vi "Test SWIR Camera.vi"(8 "error in (no error)":errorcluster) -> (0 "error out":errorcluster)   [LabVIEW 2018]
uses:
  <vilib>/vision/driver/IMAQdx.llb/IMAQdx Attribute Type.ctl
  <vilib>/vision/driver/IMAQdx.llb/IMAQdx Camera Control Mode.ctl
  82cda5bc-cbb3-4d55-9bbe-1a30e1cf78ab.vi
  <vilib>/Utility/file.llb/Write Delimited Spreadsheet (string).vi
  <vilib>/vision/driver/NI_Vision_Acquisition_Software.lvlib
  <resource>/objmgr/imaqdx.rc
panel:
  out "ValueU32":u32
  out "EnumStrings[]":string[](array[string])
  out "EnumValues[]":u32[](array[numeric])
  out "ValueString":string
  out "Array":string[](array[string])=["CameraAttributes::DeviceControl::DeviceInformationCommon::DeviceFirmwareRelease::DeviceFirmwareReleaseMajor", "CameraAttributes::DeviceControl::DeviceInformationCommon::DeviceFirmwareRelease::DeviceFirmwareReleaseMinor", "CameraAttributes::DeviceControl::DeviceInformationCommon::DeviceFirmwareRelease::DeviceFirmwareReleaseBuild", "CameraAttributes::DeviceControl::DeviceInformationCommon::DeviceApplicationRelease::DeviceAppReleaseMajor", "CameraAttributes::DeviceControl::DeviceInformationCommon::DeviceApplicationRelease::DeviceAppReleaseMinor", "CameraAttributes::DeviceControl::DeviceInformationCommon::DeviceApplicationRelease::DeviceAppReleaseBuild", "CameraAttributes::DeviceControl::DeviceInformationCommon::DeviceXMLRelease::DeviceXMLReleaseMajor", "CameraAttributes::DeviceControl::DeviceInformationCommon::DeviceXMLRelease::DeviceXMLReleaseMinor", "CameraAttributes::DeviceControl::DeviceInformationCommon::DeviceXMLRelease::DeviceXMLReleaseBuild", "AcquisitionAttributes::AdvancedEthernet::BandwidthControl::ActualPeakBandwidth", "AcquisitionAttributes::AdvancedEthernet::BandwidthControl::DesiredPeakBandwidth", "AcquisitionAttributes::AdvancedEthernet::Controller::DestinationMode", "AcquisitionAttributes::AdvancedEthernet::Controller::DestinationMulticastAddress", "AcquisitionAttributes::AdvancedEthernet::EventParameters::MaxOutstandingEvents", "AcquisitionAttributes::AdvancedEthernet::FirewallTraversal::Enabled", "AcquisitionAttributes::AdvancedEthernet::FirewallTraversal::KeepAliveTime", "AcquisitionAttributes::AdvancedEthernet::FirewallTraversal::Supported", "AcquisitionAttributes::AdvancedEthernet::ResendParameters::MaxResendsPerPacket", "AcquisitionAttributes::AdvancedEthernet::ResendParameters::MemoryWindowSize", "AcquisitionAttributes::AdvancedEthernet::ResendParameters::MissingPacketTimeout", "AcquisitionAttributes::AdvancedEthernet::ResendParameters::NewPacketTimeout", "AcquisitionAttributes::AdvancedEthernet::ResendParameters::ResendBatchingPercentage", "AcquisitionAttributes::AdvancedEthernet::ResendParameters::ResendResponseTimeout", "AcquisitionAttributes::AdvancedEthernet::ResendParameters::ResendThresholdPercentage", "AcquisitionAttributes::AdvancedEthernet::ResendParameters::ResendTimerResolution", "AcquisitionAttributes::AdvancedEthernet::ResendParameters::ResendsEnabled", "AcquisitionAttributes::AdvancedEthernet::TestPacketParameters::MaxTestPacketRetries", "AcquisitionAttributes::AdvancedEthernet::TestPacketParameters::TestPacketEnabled", "AcquisitionAttributes::AdvancedEthernet::TestPacketParameters::TestPacketTimeout", "CameraAttributes::DeviceControl::CoolingControl::CoolingMode", "CameraAttributes::DeviceControl::CoolingControl::CoolingTargetTemperature", "CameraAttributes::DeviceControl::CoolingControl::CoolingPower", "CameraAttributes::DeviceControl::CoolingControl::CoolingMaximalPower", "CameraAttributes::DeviceControl::CoolingControl::CoolingActualPower", "CameraAttributes::DeviceControl::CoolingControl::CoolingTargetTemperatureReached", "CameraAttributes::DeviceControl::DeviceInformationCommon::DeviceVendorName", "CameraAttributes::DeviceControl::DeviceInformationCommon::DeviceModelName", "CameraAttributes::DeviceControl::DeviceInformationCommon::DeviceManufacturerInfo", "CameraAttributes::DeviceControl::DeviceInformationCommon::DeviceVersion", "CameraAttributes::DeviceControl::DeviceInformationCommon::DeviceID", "CameraAttributes::DeviceControl::DeviceInformationCommon::DeviceUserID", "CameraAttributes::DeviceControl::DeviceInformationCommon::DeviceScanType", "CameraAttributes::AcquisitionControl::TriggerInControl::TriggerInMode", "CameraAttributes::AcquisitionControl::TriggerInControl::TriggerInEnable", "CameraAttributes::AcquisitionControl::TriggerInControl::TriggerInSensitivity", "CameraAttributes::AcquisitionControl::TriggerInControl::TriggerInPolarity", "CameraAttributes::AcquisitionControl::TriggerInControl::TriggerInDelay", "CameraAttributes::AcquisitionControl::TriggerInControl::TriggerInSkip", "CameraAttributes::AcquisitionControl::TriggerOutControl::TriggerOutEnable", "CameraAttributes::AcquisitionControl::TriggerOutControl::TriggerOutSource", "CameraAttributes::AcquisitionControl::TriggerOutControl::TriggerOutPolarity", "CameraAttributes::AcquisitionControl::TriggerOutControl::TriggerOutDelay", "CameraAttributes::AcquisitionControl::TriggerOutControl::TriggerOutWidth", "CameraAttributes::ImageProcessingControl::AutoGainControl::OffsetControl", "CameraAttributes::ImageProcessingControl::AutoGainControl::GainControl", "CameraAttributes::ImageProcessingControl::AutoGainControl::AutoModeUpdate", "CameraAttributes::ImageProcessingControl::AutoGainControl::OffsetUsed", "CameraAttributes::ImageProcessingControl::AutoGainControl::GainUsed", "CameraAttributes::ImageProcessingControl::AutoGainControl::ManualModeControl::ManualModeOffset", "CameraAttributes::ImageProcessingControl::AutoGainControl::ManualModeControl::ManualModeGain", "CameraAttributes::ImageProcessingControl::AutoGainControl::AutoModeControl::AutoModeOutputHistogramMidpoint", "CameraAttributes::ImageProcessingControl::AutoGainControl::AutoModeControl::AutoModeMaximalGain", "CameraAttributes::ImageProcessingControl::AutoGainControl::AutoModeControl::AutoModeRegulationSpeed", "CameraAttributes::ImageProcessingControl::AutoGainControl::OutliersControl::OutliersExpressedAs", "CameraAttributes::ImageProcessingControl::AutoGainControl::OutliersControl::OutliersDark", "CameraAttributes::ImageProcessingControl::AutoGainControl::OutliersControl::OutliersBright", "CameraAttributes::ImageProcessingControl::AutoGainControl::OutliersControl::OutliersBrightDisplayColor", "CameraAttributes::ImageProcessingControl::AutoGainControl::InputHistogramControl::InputHistogramBegin", "CameraAttributes::ImageProcessingControl::AutoGainControl::InputHistogramControl::InputHistogramMidpoint", "CameraAttributes::ImageProcessingControl::AutoGainControl::InputHistogramControl::InputHistogramEnd", "CameraAttributes::TransportLayer::GevVersion::GevVersionMajor", "CameraAttributes::TransportLayer::GevVersion::GevVersionMinor", "CameraAttributes::TransportLayer::GevMACAddress::GevMACAddressHigh", "CameraAttributes::TransportLayer::GevMACAddress::GevMACAddressLow", "CameraAttributes::TransportLayer::GevTimestamp::GevTimestampTickFrequency", "CameraAttributes::TransportLayer::GevTimestamp::GevTimestampControl::GevTimestampControlReset", "AcquisitionAttributes::AdvancedEthernet::GigEDriverType", "AcquisitionAttributes::AdvancedGenicam::CommandTimeout", "AcquisitionAttributes::AdvancedGenicam::EventsEnabled", "AcquisitionAttributes::AdvancedGenicam::EventsSupported", "AcquisitionAttributes::AdvancedGenicam::IgnoreCameraValidationErrors", "AcquisitionAttributes::Bayer::Algorithm", "AcquisitionAttributes::Bayer::GainB", "AcquisitionAttributes::Bayer::GainG", "AcquisitionAttributes::Bayer::GainR", "AcquisitionAttributes::Bayer::Pattern", "AcquisitionAttributes::ChunkDataDecoding::ChunkDataDecodingEnabled", "AcquisitionAttributes::ChunkDataDecoding::MaximumChunkCopySize", "CameraAttributes::DeviceControl::DeviceVTestGVoltage", "CameraAttributes::DeviceControl::DeviceDetSubVoltage", "CameraAttributes::DeviceControl::DeviceVcmVoltage", "CameraAttributes::DeviceControl::DeviceCtiaRefVoltage", "CameraAttributes::DeviceControl::DeviceROICBiasCurrent", "CameraAttributes::DeviceControl::DeviceGain", "CameraAttributes::DeviceControl::DeviceTemperature", "CameraAttributes::DeviceControl::DeviceBoardTemperature", "CameraAttributes::AcquisitionControl::AcquisitionMode", "CameraAttributes::AcquisitionControl::ExposureTimeAbs", "CameraAttributes::AcquisitionControl::IntegrationMode", "CameraAttributes::AcquisitionControl::MinimumFrameTime", "CameraAttributes::AcquisitionControl::SoftwareTrigger", "CameraAttributes::AcquisitionControl::TriggerDirection", "CameraAttributes::ImageFormatControl::WidthMax", "CameraAttributes::ImageFormatControl::HeightMax", "CameraAttributes::ImageFormatControl::Width", "CameraAttributes::ImageFormatControl::Height", "CameraAttributes::ImageFormatControl::OffsetX", "CameraAttributes::ImageFormatControl::OffsetY", "CameraAttributes::ImageFormatControl::ReverseX", "CameraAttributes::ImageFormatControl::ReverseY", "CameraAttributes::ImageFormatControl::PixelFormat", "CameraAttributes::ImageFormatControl::FooterEnable", "CameraAttributes::ImageCorrectionControl::RawMode", "CameraAttributes::ImageCorrectionControl::FPNCorrection", "CameraAttributes::ImageCorrectionControl::PRNUCorrection", "CameraAttributes::ImageCorrectionControl::BPRCorrection", "CameraAttributes::ImageCorrectionControl::ImageCorrectionBlackClip", "CameraAttributes::ImageCorrectionControl::ImageCorrectionWhiteClip", "CameraAttributes::UserSetControl::UserSetSelector", "CameraAttributes::UserSetControl::UserSetLoad", "CameraAttributes::UserSetControl::UserSetSave", "CameraAttributes::UserSetControl::UserSetDefaultSelector", "CameraAttributes::UserSetControl::UserSetCurrent", "CameraAttributes::TransportLayer::PayloadSize", "CameraAttributes::TransportLayer::GevLinkSpeed", "CameraAttributes::TransportLayer::GevLinkSpeedSelection", "AcquisitionAttributes::BitsPerPixel", "AcquisitionAttributes::HardwareMaximumQueuedBufferCount", "AcquisitionAttributes::HardwareRequeueBufferListThreshold", "AcquisitionAttributes::ImageDecoderCopyMode", "AcquisitionAttributes::IncompleteBufferMode", "AcquisitionAttributes::OutputImageType", "AcquisitionAttributes::OverwriteMode", "AcquisitionAttributes::PacketSize", "AcquisitionAttributes::ReceiveTimestampMode", "AcquisitionAttributes::ShiftPixelBits", "AcquisitionAttributes::SwapPixelBytes", "AcquisitionAttributes::Timeout", "CameraInformation::BaseAddress", "CameraInformation::BusType", "CameraInformation::HostIPAddress", "CameraInformation::HostMACAddress", "CameraInformation::HostNetworkInterfaceName", "CameraInformation::IPAddress", "CameraInformation::ModelName", "CameraInformation::PrimaryURLString", "CameraInformation::SecondaryURLString", "CameraInformation::SerialNumberHigh", "CameraInformation::SerialNumberLow", "CameraInformation::VendorName", "StatusInformation::AcqInProgress", "StatusInformation::HandledEventCount", "StatusInformation::IncompleteBufferCount", "StatusInformation::LastBufferCount", "StatusInformation::LastBufferNumber", "StatusInformation::LostBufferCount", "StatusInformation::LostEventCount", "StatusInformation::LostPacketCount", "StatusInformation::ReceivedResendPackets", "StatusInformation::RequestedResendPacketCount"]
  out "Attribute Information Array":T2(array[cluster])
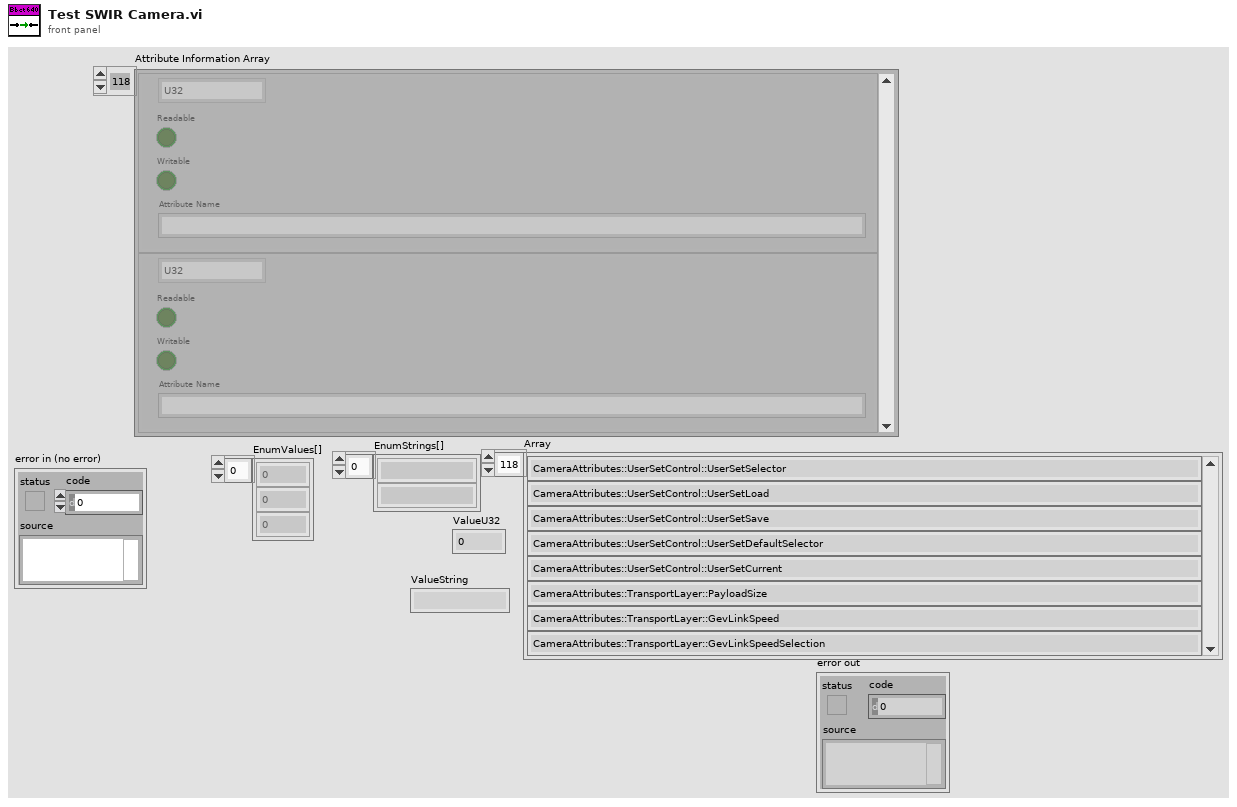
[diagram p1: front panel]
types:
  T1 = typedef "NI_Vision_Acquisition_Software.lvlib/IMAQdx Attribute Type.ctl" = enum32{"U32", "I64", "DBL", "String", "Enum", "Bool", "Command"}
  T2 = cluster{"Attribute Type":T1, "Readable":bool, "Writable":bool, "Attribute Name":string}[]
  T3 = typedef "NI_Vision_Acquisition_Software.lvlib/IMAQdx Camera Control Mode.ctl" = enum32{"Controller", "Listener"}
  T4 = typedef "IMAQdx.ctl" = refnum<k21>
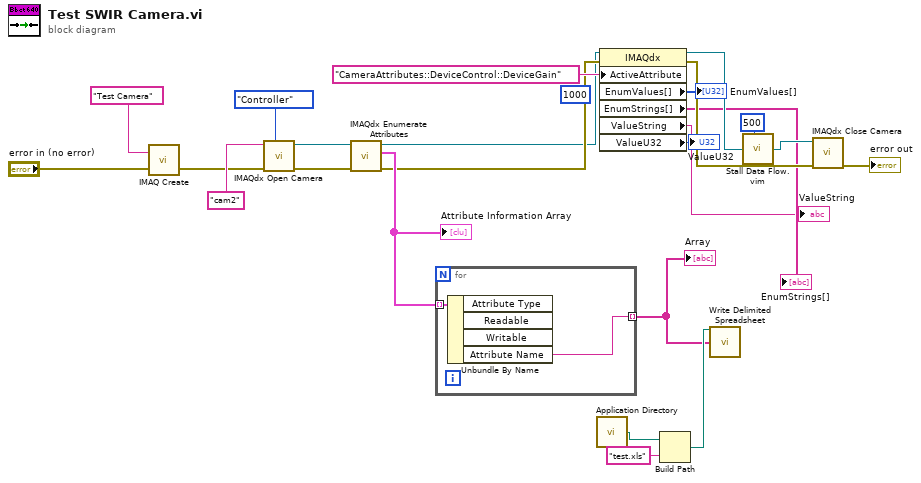
[diagram p0: block diagram]
diagram:
  (unwired) i64 1000 ("ValueI64")
  n1 = call "IMAQ Create"("Image Name"="Test Camera", "error in (no error)"="error in (no error)") -> ("error out"=w20:errorcluster)  [unwired: 3 in, 1 out]
  n2 = call <vilib>:"IMAQdx Open Camera.vi"("Camera Control Mode"=IMAQdx_Camera_Control_Mode."Controller", "error in"=w20, "Session In"="cam2") -> ("error out"=w19:errorcluster, "Session Out"=w13:T4)  [unwired: 7 in]
  n3 = call <vilib>:"IMAQdx Enumerate Attributes.vi"("error in"=w19, "Session In"=w13) -> ("error out"=w11:errorcluster, "Attribute Information Array"=w18:T2, "Session Out"=w8:T4)  [unwired: 7 in]
  "Attribute Information Array" <- w18
  n4 = for {
    tunnel: w18 -> [w26] mode=indexing
    tunnel: [w25] -> w14 mode=indexing
    n5 = Unbundle By Name(w26) -> ("Attribute Name"=w25:string)  [unwired: 3 out]
  }
  "Array" <- w14
  n6 = call <vilib>:"Application Directory.vi"() -> ("Application Directory"=w17:path)
  n7 = property class="IMAQdx"(reference=w8, error in=w11, "ActiveAttribute"="CameraAttributes::DeviceControl::DeviceGain") -> (reference out=w7:T4, error out=w9:errorcluster, "EnumValues[]"=→"EnumValues[]":u32[], "EnumStrings[]"=→"EnumStrings[]":string[], "ValueString"=→"ValueString":string, "ValueU32"=→"ValueU32":u32)
  n8 = Build Path(base path=w17, name or relative path="test.xls") -> (appended path=w15:path)
  n9 = call-poly <vilib>:"Write Delimited Spreadsheet.vi"("file path (dialog if empty)"=w15, "1D data"=w14) -> ()  [unwired: 12 in, 2 out]
  n10 = call "Stall Data Flow.vim"("value in"=w7, "milliseconds to wait"=u32 500) -> ("value out"=w6:T4)  [unwired: 1 out]
  n11 = call <vilib>:"IMAQdx Close Camera.vi"("error in"=w9, "Session In"=w6) -> ("error out"=→"error out":errorcluster)  [unwired: 9 in]
